vi "serial_mvmnt_1step_2.vi"(2 "Conn. Axes":string[](array[string]), 3 "error in":errorcluster, 4 "Z step":dbl, 5 "System no.":i32) -> (0 "error out":errorcluster, 1 "Position":dbl)   [LabVIEW 2016]
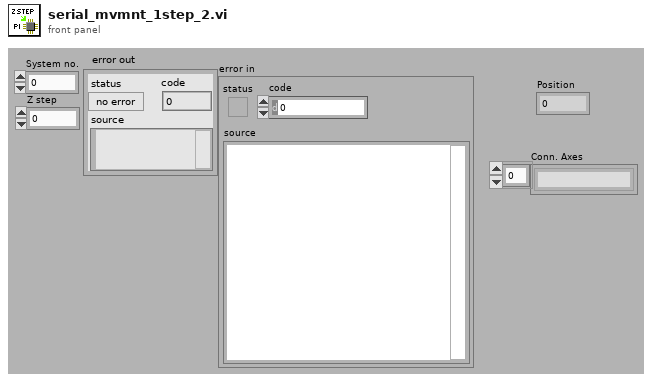
[diagram p1: front panel]
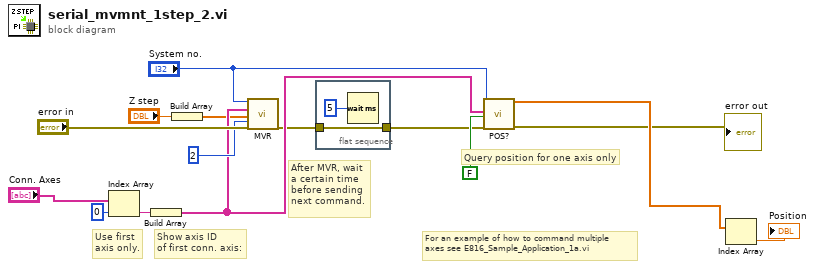
[diagram p0: block diagram]
diagram:
  # "Show axis ID\nof first conn. axis:"
  # "For an example of how to command multiple\naxes see E816_Sample_Application_1a.vi"
  # "Use first\naxis only."
  # "After MVR, wait\na certain time\nbefore sending\nnext command."
  # "Query position for one axis only"
  n1 = Index Array(array="Conn. Axes", index=0) -> (element=w9:string)
  n2 = Build Array(w9) -> (w8:string[])
  n3 = Build Array("Z step") -> (w6:dbl[])
  n4 = call "MVR.vi"("System no."="System no.", "Axes to move"=w8, "Position values"=w6, "No.of digits"=i16 2, "error in"="error in") -> ("error out"=w1:errorcluster)  [unwired: 14 out]
  n5 = flat-sequence {
    tunnel: w1 -> [w17]
    tunnel: [w17] -> w2
    frame #0 {
      n6 = Wait (ms)(milliseconds to wait=u32 5) -> ()  [unwired: 1 out]
    }
  }
  n7 = call "POS?.vi"("System no."="System no.", "Axes to query"=w8, "All axes?"=FALSE, "error in"=w2) -> ("Position"=w5:dbl[], "error out"=→"error out":errorcluster)  [unwired: 1 in, 13 out]
  n8 = Index Array(array=w5) -> (element=→"Position":dbl)  [unwired: 1 in]
